vi "Autonomous A3 Right-deliverswitch-move out of way.vi"   [LabVIEW 2017]
uses:
  Framework/Robot Global Data.vi
types:
  T1 = typedef "Command Status Info.ctl" = cluster{"Name":string, "Status":T2, "notifier out":T3}
  T2 = typedef "Completion Status.ctl" = enum16{"Successful", "Aborted", "Incomplete"}
  T3 = typedef "Completion Notifier.ctl" = refnum<notifier>
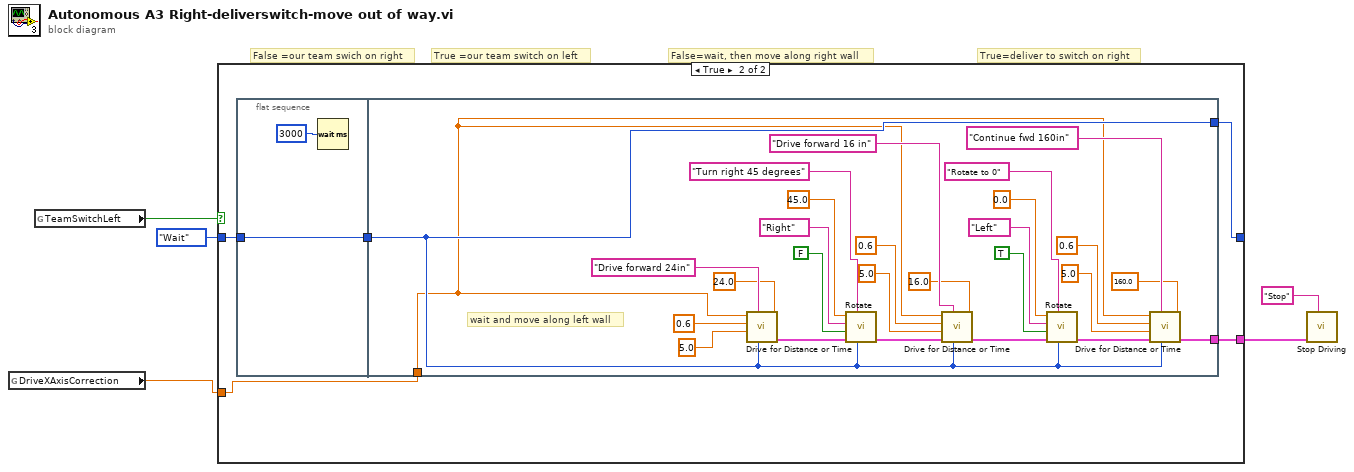
[diagram p0: block diagram]
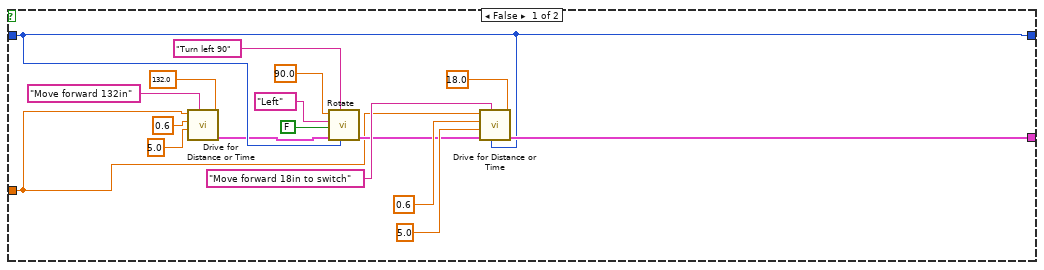
[diagram p2: hidden frame]
diagram:
  # "False=wait, then move along right wall"
  # "True=deliver to switch on right"
  # "False =our team swich on right"
  # "True =our team switch on left"
  n1 = global read "Robot Global Data.vi" "DriveXAxisCorrection"() -> (w1:dbl)
  n2 = global read "Robot Global Data.vi" "TeamSwitchLeft"() -> (w2:bool)
  n3 = case shown="True" w2 {
    tunnel: [w17 w27] -> w4
    tunnel: [w16 w24] -> _
    tunnel: enum16{"Start", "Wait"}."Wait" ("Synchronication") -> [w16 w26]
    tunnel: w1 -> [w6 w23]
    frame False {
      n4 = call "Drive for Distance or Time.vi"("Distance (inches)"=132.0, "Description"="Move forward 132in", "Seconds"=5.0, "Y-axis"=0.6 ("Right Speed"), "X-axis"=w6) -> ("Command Info Out"=w7:T1)  [unwired: 6 in]
      n5 = call "Rotate.vi"("Synchronication"=w16, "Description"="Turn left 90", "Command Info In"=w7, "Force Degrees"=FALSE, "Turn Direction"="Left" ("Direction"), "Degrees"=90.0 ("Seconds")) -> ("Command Info Out"=w18:T1)  [unwired: 5 in]
      n6 = call "Drive for Distance or Time.vi"("Distance (inches)"=18.0, "Synchronication"=w16, "Description"="Move forward 18in to switch", "Command Info In"=w18, "Seconds"=5.0, "Y-axis"=0.6 ("Right Speed"), "X-axis"=w6) -> ("Command Info Out"=w17:T1)  [unwired: 4 in]
    }
    frame True {
      n7 = flat-sequence {
        tunnel: w26 -> [w29]
        tunnel: [w29] -> w25
        tunnel: [w42] -> w27
        tunnel: w25 -> [w40]
        tunnel: [w40] -> w24
        tunnel: w23 -> [w30]
        frame #0 {
          n8 = Wait (ms)(milliseconds to wait=u32 3000) -> ()  [unwired: 1 out]
        }
        frame #1 {
          # "wait and move along left wall"
          n9 = call "Drive for Distance or Time.vi"("Distance (inches)"=24.0, "Synchronication"=w40, "Description"="Drive forward 24in", "Seconds"=5.0, "Y-axis"=0.6 ("Right Speed"), "X-axis"=w30) -> ("Command Info Out"=w55:T1)  [unwired: 5 in]
          n10 = call "Rotate.vi"("Synchronication"=w40, "Description"="Turn right 45 degrees", "Command Info In"=w55, "Force Degrees"=FALSE, "Turn Direction"="Right" ("Direction"), "Degrees"=45.0 ("Seconds")) -> ("Command Info Out"=w53:T1)  [unwired: 5 in]
          n11 = call "Drive for Distance or Time.vi"("Distance (inches)"=16.0, "Synchronication"=w40, "Description"="Drive forward 16 in", "Command Info In"=w53, "Seconds"=5.0, "Y-axis"=0.6 ("Right Speed"), "X-axis"=w30) -> ("Command Info Out"=w52:T1)  [unwired: 4 in]
          n12 = call "Rotate.vi"("Synchronication"=w40, "Description"="Rotate to 0", "Command Info In"=w52, "Force Degrees"=TRUE, "Turn Direction"="Left" ("Direction"), "Degrees"=0.0 ("Left Speed")) -> ("Command Info Out"=w43:T1)  [unwired: 5 in]
          n13 = call "Drive for Distance or Time.vi"("Distance (inches)"=160.0, "Synchronication"=w40, "Description"="Continue fwd 160in", "Command Info In"=w43, "Seconds"=5.0, "Y-axis"=0.6 ("Right Speed"), "X-axis"=w30) -> ("Command Info Out"=w42:T1)  [unwired: 4 in]
        }
      }
    }
  }
  n14 = call "Stop Driving.vi"("Description"="Stop", "Command Info In"=w4) -> ()  [unwired: 9 in, 1 out]
